vi "bitsOperator.vi"(0 "b":u8 format="%b", 1 "bitStart":u8, 2 "length":u8, 3 "data":u8 format="%b") -> (7 "x .or. y?":u8 format="%b")   [LabVIEW 2016]
panel:
  out "x << y":u8 format="%b"
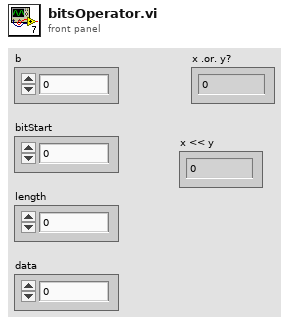
[diagram p1: front panel]
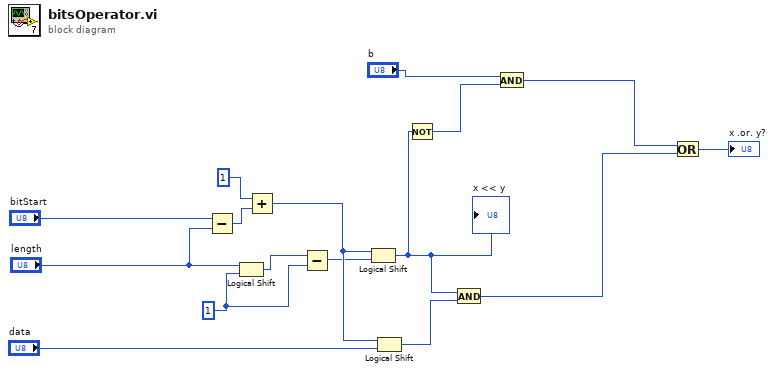
[diagram p0: block diagram]
diagram:
  w1 = u8 1 ("x")
  n1 = Subtract(x="bitStart", y="length") -> (x-y=w6:u8)
  n2 = Logical Shift(y="length", x=w1) -> (x << y=w2:u8)
  n3 = Add(x=u8 1, y=w6) -> (x+y=w8:u8)
  n4 = Subtract(x=w2, y=w1) -> (x-y=w3:u8)
  n5 = Logical Shift(y=w8, x=w3) -> (x << y=w11:u8)
  "x << y" <- w11
  n6 = Logical Shift(y=w8, x="data") -> (x << y=w10:u8)
  n7 = Not(x=w11) -> (.not. x?=w12:u8)
  n8 = And(x=w11, y=w10) -> (x .and. y?=w15:u8)
  n9 = And(x="b", y=w12) -> (x .and. y?=w14:u8)
  n10 = Or(x=w14, y=w15) -> (x .or. y?=→"x .or. y?":u8)
